vi "Hardware-DIScope-Snapshot.vi"(4 "Snapshot":bool, 6 "File name or relative path":string, 8 "Channels":T1, 9 "dT [s]":sgl format="%#_6p", 10 "New Data":bool, 11 "Data":sgl[][](array[numeric])) -> ()   [LabVIEW 2016, in "DSI-RT.lvlib"]
uses:
  DSI-RT.lvlib
  <vilib>/Powertrain Controls/Device Drivers/DCM/Rev0/RT/DI - ADC Select.ctl
  <vilib>/Powertrain Controls/Device Drivers/DCM/Rev0/FPGA/DI - ADC Signals.ctl
  <vilib>/Powertrain Controls/Device Drivers/DCM/Rev0/FPGA/DCM - FPGA.lvlib
  <vilib>/Powertrain Controls/Device Drivers/DCM/Rev0/RT/DCM - RT.lvclass
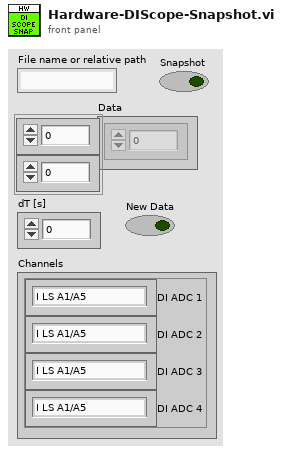
[diagram p1: front panel]
types:
  T1 = typedef "DCM - RT.lvclass/DI - ADC Select.ctl" = cluster{"DI ADC 1":T2, "DI ADC 2":T2, "DI ADC 3":T2, "DI ADC 4":T2}
  T2 = typedef "DCM - FPGA.lvlib/DI - ADC Signals.ctl" = enum8{"I LS A1/A5", "I LS A2/A6", "I LS A3/A7", "I LS A4", "I LS A8/PumpA", "V PZ A1", "V PZ A2", "V PZ A3", "V PZ A4", "V S A1", "V S A2", "V S A3", "V S A4", "V S A5", "V S A6", "V S A7", "V S A8", "V Pump A", "V Secondary A1A2", "V Secondary A3A4", "V Ext HV A", "------------------------ ", "I LS B1/B5", "I LS B2/B6", "I LS B3/B7", "I LS B4", "I LS B8/PumpB", "V PZ B1", "V PZ B2", "V PZ B3", "V PZ B4", "V S B1", "V S B2", "V S B3", "V S B4", "V S B5", "V S B6", "V S B7", "V S B8", "V Pump B", "V Secondary B1B2", "V Secondary B3B4", "V Ext HV B", "-------------------------  ", "AI 1", "AI 2", "AI 3", "AI 4", "AI 5", "AI 6", "AI 7", "AI 8", "AI 9", "AI 10", "AI 11", "AI 12", "-------------------------   ", "V DRVP"}
  T3 = enum16{"open", "open or create", "create or replace", "create", "open (read-only)"}
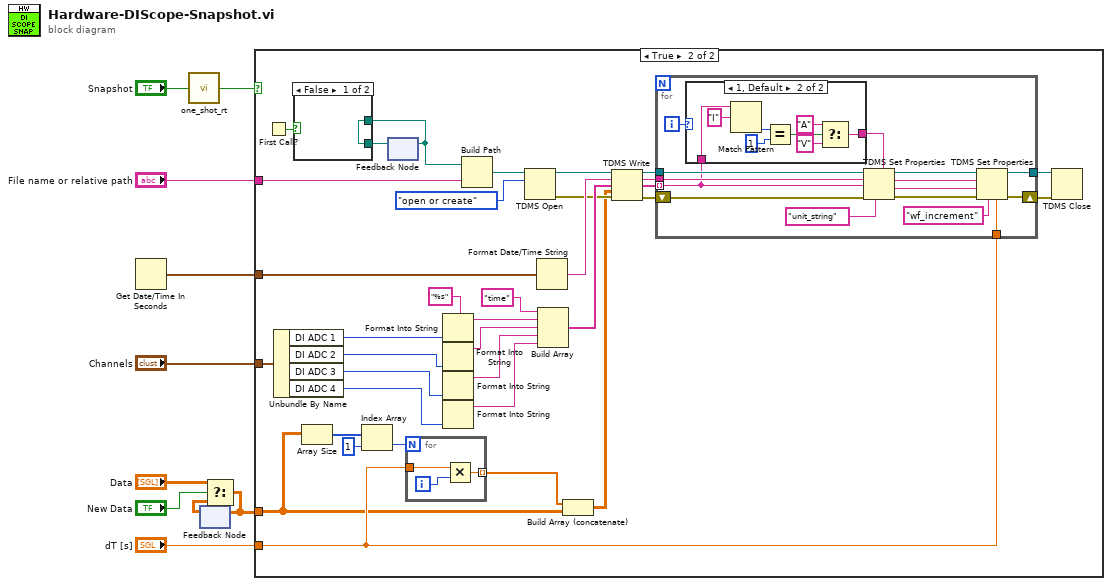
[diagram p0: block diagram]
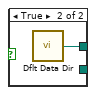
[diagram p3: hidden frame]
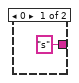
[diagram p4: hidden frame]
diagram:
  n1 = Get Date/Time In Seconds() -> (seconds since 1Jan1904=w7:timestamp)
  n2 = call <vilib>:"one_shot_rt.vi"("I"="Snapshot") -> ("O"=w1:bool)
  n3 = feedback #1() -> (w6:sgl[][])  [unwired: 1 in]
  n4 = Select(t="Data", s="New Data", f=w6) -> (s? t:f=w4:sgl[][])
  n5 = feedback-in #1(w4) -> ()
  n6 = case shown="True" w1 {
    tunnel: "File name or relative path" -> [_ w45]
    tunnel: "dT [s]" -> [_ w20]
    tunnel: "Channels" -> [_ w44]
    tunnel: w7 -> [_ w43]
    tunnel: w4 -> [_ w19]
    frame False {
    }
    frame True {
      w40 = "%s" ("format string")
      n7 = First Call?() -> (First Call?: T/F=w41:bool)
      n8 = Unbundle By Name(w44) -> ("DI ADC 1"=w39:T2, "DI ADC 2"=w38:T2, "DI ADC 3"=w37:T2, "DI ADC 4"=w36:T2)
      n9 = Array Size(array=w19) -> (size(s)=w21:i32[])
      n10 = Index Array(array=w21, index=1) -> (element=w18:i32)
      n11 = feedback #2() -> (w14:path)  [unwired: 1 in]
      n12 = case shown="False" w41 {
        tunnel: [w46 w47] -> w13
        tunnel: w14 -> [w46 _]
        frame False {
        }
        frame True {
          n13 = call <vilib>:"Dflt Data Dir.vi"() -> ("App:Default Data Directory"=w47:path)
        }
      }
      n14 = feedback-in #2(w13) -> ()
      n15 = for {
        N: w18 -> [_]
        tunnel: w20 -> [w73]
        tunnel: [w72] -> w16 mode=indexing
        i -> [w74]
        n16 = Multiply(x=w73, y=w74) -> (x*y=w72:sgl)
      }
      n17 = Format Into String(format string=w40, w39) -> (resulting string=w35:string)  [unwired: 2 in, 1 out]
      n18 = Format Into String(format string=w40, w38) -> (resulting string=w34:string)  [unwired: 2 in, 1 out]
      n19 = Format Into String(format string=w40, w37) -> (resulting string=w32:string)  [unwired: 2 in, 1 out]
      n20 = Format Into String(format string=w40, w36) -> (resulting string=w33:string)  [unwired: 2 in, 1 out]
      n21 = Build Path(base path=w13, name or relative path=w45) -> (appended path=w12:path)
      n22 = TDMS Open(10:T3."open or create" ("operation (0:open)"), 11:w12) -> (0:w25:errorcluster, 3:w42:refnum<k34>)  [unwired: 5 in]
      n23 = Format Date/Time String(seconds (now)=w43) -> (date/time string=w31:string)  [unwired: 2 in]
      n24 = Build Array("time" ("element"), w35, w34, w32, w33) -> (w26:string[])
      n25 = Build Array (concatenate)(w16, w19) -> (w22:sgl[][])
      n26 = TDMS Write(0:w42, 5:w31, 7:w26, 9:w22, 11:w25) -> (4:w30:refnum<k34>, 6:w29:string, 8:w28:string[], 15:w24:errorcluster)  [unwired: 1 in]
      n27 = for {
        tunnel: w30 -> [w62]
        tunnel: w29 -> [w61]
        tunnel: w28 -> [w60] mode=indexing
        tunnel: [w53] -> w27
        shift-right: [w54] -> w23
        shift-left: w24 -> [w57]
        tunnel: w20 -> [w49]
        i -> [w48]
        n28 = case shown="1, Default" w48 {
          tunnel: w60 -> [_ w68]
          tunnel: ["s" ("regular expression") w67] -> w59
          frame 0 {
          }
          frame 1, Default {
            n29 = Match Pattern(string=w68, regular expression="I") -> (offset past match=w66:i32)  [unwired: 1 in, 3 out]
            n30 = Equal?(x=w66, y=1) -> (x = y?=w64:bool)
            n31 = Select(t="A" ("regular expression"), s=w64, f="V" ("regular expression")) -> (s? t:f=w67:string)
          }
        }
        n32 = TDMS Set Properties(5:w59, 7:"unit_string", 8:w57, 9:w60, 10:w61, 11:w62) -> (0:w55:errorcluster, 1:w51:string, 2:w52:string, 3:w56:refnum<k34>)
        n33 = TDMS Set Properties(5:w49, 7:"wf_increment" ("String"), 8:w55, 9:w51, 10:w52, 11:w56) -> (0:w54:errorcluster, 3:w53:refnum<k34>)  [unwired: 2 out]
      }
      n34 = TDMS Close(8:w23, 11:w27) -> ()  [unwired: 2 out]
    }
  }
